vi "Zstack.vi"(0 "Total DataPoints":i32, 1 "Datapoint Index within Path":i32, 2 "Current Position":dbl, 3 "Input Position":dbl, 4 "A/D Rate":dbl) -> (14 "Calculated Position":dbl)   [LabVIEW 2012]
panel:
  # "Nano-Route™ 3D"
  # "Custom Path Generating SubVI"
  # "Standard Inputs"
  # "Required Output"
  # "Custom Inputs"
  # "Custom Outputs"
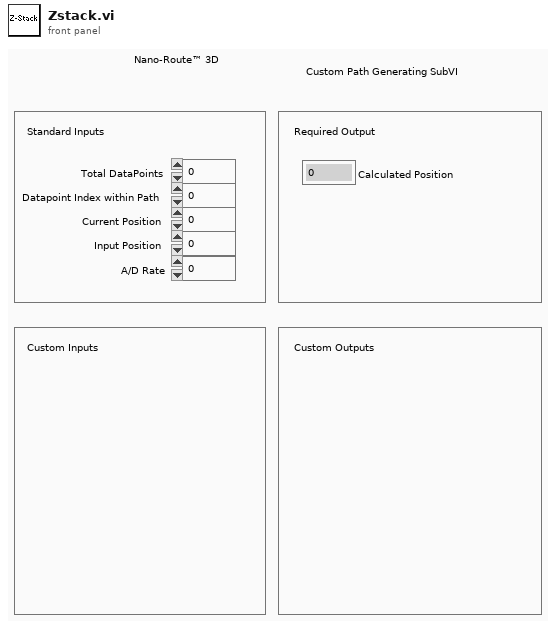
[diagram p1: front panel]
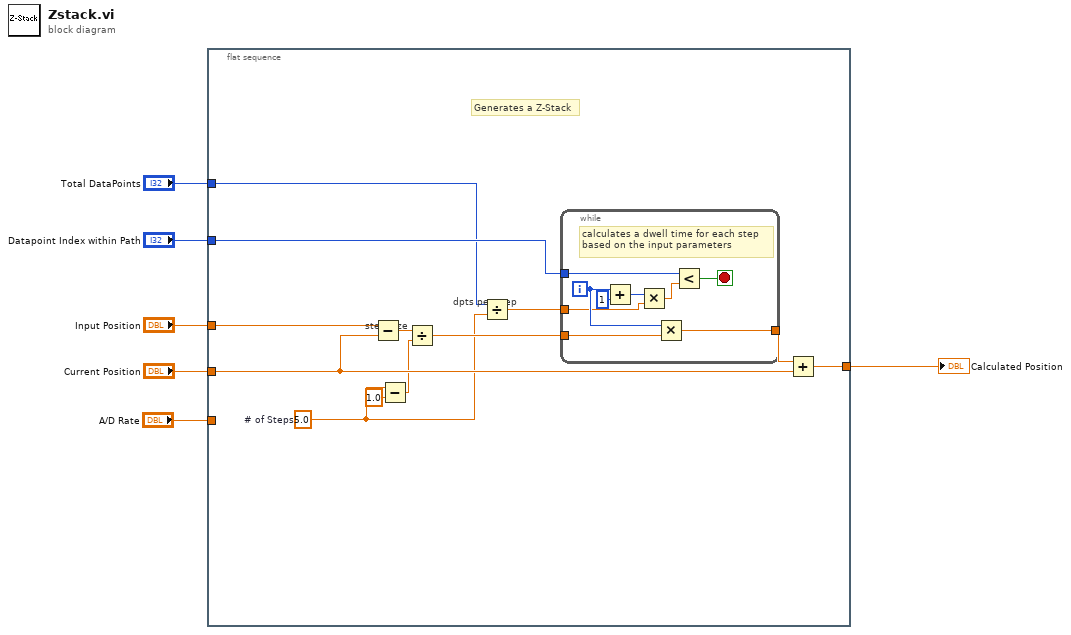
[diagram p0: block diagram]
diagram:
  n1 = flat-sequence {
    tunnel: "Input Position" -> [w15]
    tunnel: "Total DataPoints" -> [w10]
    tunnel: "Datapoint Index within Path" -> [w17]
    tunnel: "Current Position" -> [w14]
    tunnel: [w18] -> w2
    tunnel: "A/D Rate" -> [_]
    frame #0 {
      w8 = 5.0  # # of Steps
      # "dpts per step"
      # "step size"
      # "Generates a Z-Stack"
      n2 = Subtract(x=w15, y=w14) -> (x-y=w16:dbl)
      n3 = Subtract(x=w8, y=1.0) -> (x-y=w9:dbl)
      n4 = Divide(x=w16, y=w9) -> (x/y=w13:dbl)
      n5 = Divide(x=w10, y=w8) -> (x/y=w11:dbl)
      n6 = while {
        tunnel: [w20] -> w12
        tunnel: w17 -> [w24]
        tunnel: w13 -> [w22]
        tunnel: w11 -> [w19]
        i -> [w21]
        stop <- w23 stop-if-true
        # "calculates a dwell time for each step\nbased on the input parameters"
        n7 = Add(x=w21, y=1) -> (x+y=w26:i32)
        n8 = Multiply(x=w26, y=w19) -> (x*y=w25:dbl)
        n9 = Multiply(x=w21, y=w22) -> (x*y=w20:dbl)
        n10 = Less?(x=w24, y=w25) -> (x < y?=w23:bool)
      }
      n11 = Add(x=w12, y=w14) -> (x+y=w18:dbl)
    }
  }
  "Calculated Position" <- w2
